vi "Untitled 1.vi"() -> ()   [LabVIEW 2024]
panel:
  in  "All?":bool
  in  "Run Selection Listbox":i32(listbox)
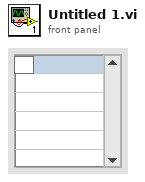
[diagram p1: front panel]
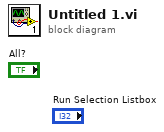
[diagram p0: block diagram]
diagram:
